vi "optogeneticsSplitList.vi"(1 "max":i32=100, 2 "delimiter":string=":", 3 "list":string) -> (0 "output":i32[](array[numeric]))   [LabVIEW 2017]
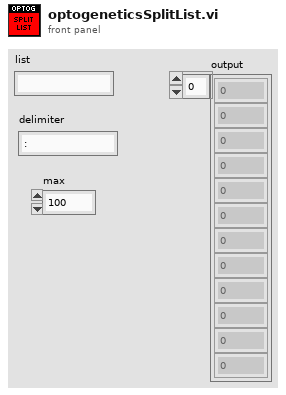
[diagram p1: front panel]
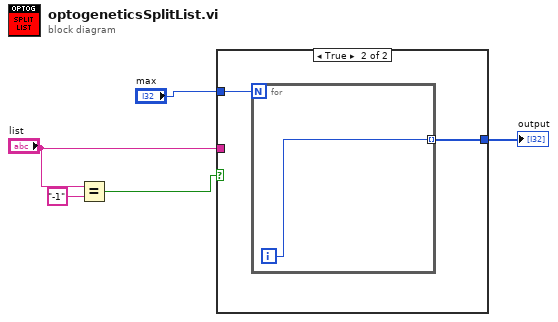
[diagram p0: block diagram]
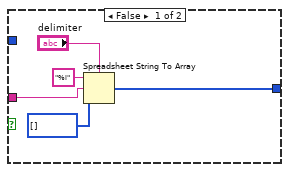
[diagram p2: hidden frame]
diagram:
  n1 = Equal?(x="list", y="-1") -> (x = y?=w3:bool)
  n2 = case shown="True" w3 {
    tunnel: "list" -> [w7 _]
    tunnel: "max" -> [_ w12]
    tunnel: [w6 w11] -> w1
    frame False {
      n3 = Spreadsheet String To Array(delimiter (Tab)="delimiter", format string="%i", spreadsheet string=w7, array type (2D Dbl)=i32[] []) -> (array=w6:i32[])
    }
    frame True {
      n4 = for {
        N: w12 -> [_]
        tunnel: [w13] -> w11 mode=indexing
        i -> [w13]
      }
    }
  }
  "output" <- w1
